vi "binary-block-to-i16.vi"(1 "Binary Block":string) -> (0 "i16 Array":i32[](array[numeric]))   [LabVIEW 2014]
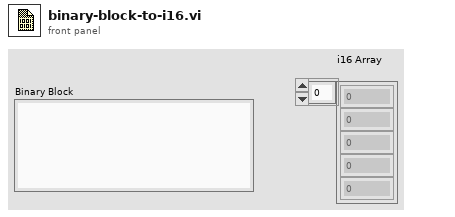
[diagram p1: front panel]
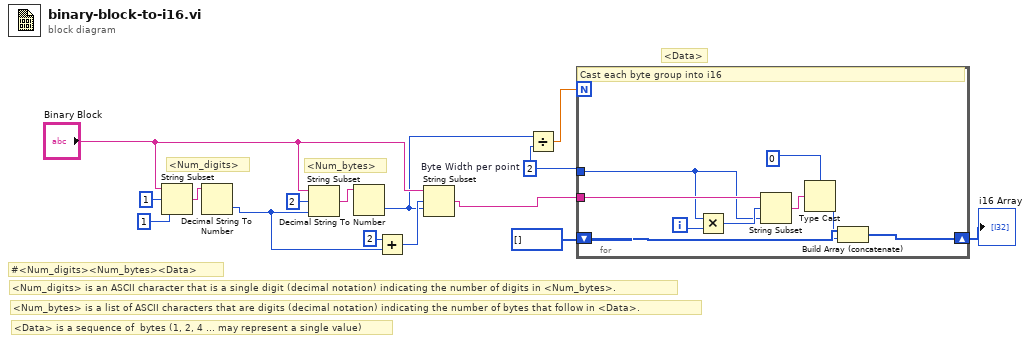
[diagram p0: block diagram]
diagram:
  w1 = u8 2  # Byte Width per point
  # "<Data>"
  # "<Num_bytes>"
  # "<Num_digits>"
  # "<Data> is a sequence of  bytes (1, 2, 4 ... may represent a single value)"
  # "<Num_bytes> is a list of ASCII characters that are digits (decimal notation) indicating the number of bytes that follow in <Data>."
  # "<Num_digits> is an ASCII character that is a single digit (decimal notation) indicating the number of digits in <Num_bytes>."
  # "#<Num_digits><Num_bytes><Data>"
  n1 = String Subset(string="Binary Block", offset (0)=1, length (rest)=1 ("length (rest)")) -> (substring=w13:string)
  n2 = Decimal String To Number(string=w13) -> (number=w10:i32)  [unwired: 2 in, 1 out]
  n3 = String Subset(string="Binary Block", offset (0)=2, length (rest)=w10) -> (substring=w8:string)
  n4 = Decimal String To Number(string=w8) -> (number=w2:i32)  [unwired: 2 in, 1 out]
  n5 = Add(x=2 ("offset (0)"), y=w10) -> (x+y=w5:i32)
  n6 = String Subset(string="Binary Block", offset (0)=w5, length (rest)=w2) -> (substring=w7:string)
  n7 = Divide(x=w2, y=w1) -> (x/y=w3:dbl)
  n8 = for {
    N: w3 -> [_]
    tunnel: w7 -> [w24]
    shift-right: [w21] -> w4
    shift-left: i32[] [] -> [w17]
    tunnel: w1 -> [w18]
    i -> [w23]
    # "Cast each byte group into i16"
    n9 = Multiply(x=w18, y=w23) -> (x*y=w22:i32)
    n10 = String Subset(string=w24, offset (0)=w22, length (rest)=w18) -> (substring=w20:string)
    n11 = Type Cast(type=i16 0, x=w20) -> (*(type *) &x=w16:i16)
    n12 = Build Array (concatenate)(w17, w16) -> (w21:i32[])
  }
  "i16 Array" <- w4
